vi "Update Method Accessors.vi"(8 "error in (no error)":errorcluster, 10 "RPC Method Parameters":T1, 11 "Server class in":refnum<vi>) -> (0 "error out":errorcluster, 3 "Server class out":refnum<vi>)   [LabVIEW 2019, in "gRPC Scripting Tools.lvlib"]
uses:
  gRPC Scripting Tools.lvlib
  TypeDefs/RPC Method Parameters.ctl
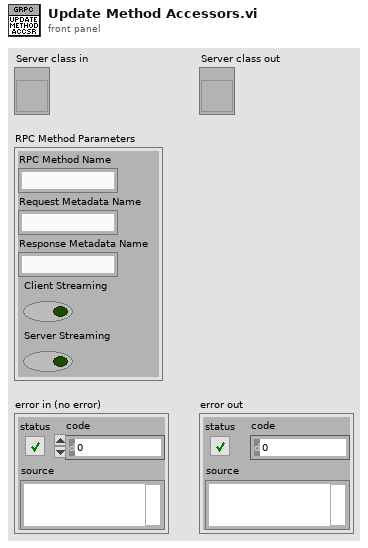
[diagram p1: front panel]
types:
  T1 = typedef "gRPC Scripting Tools.lvlib/RPC Method Parameters.ctl" = cluster{"RPC Method Name":string, "Request Metadata Name":string, "Response Metadata Name":string, "Client Streaming":bool, "Server Streaming":bool}
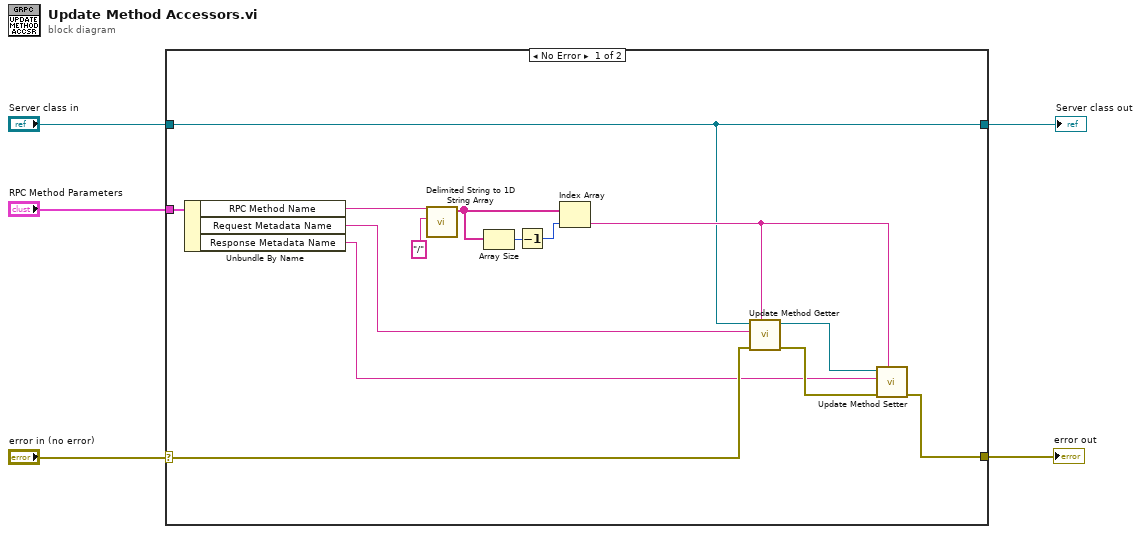
[diagram p0: block diagram]
diagram:
  n1 = case shown="No Error" "error in (no error)" {
    selector: "error in (no error)" -> [w12 w20]
    tunnel: "RPC Method Parameters" -> [w19 _]
    tunnel: "Server class in" -> [w6 w21]
    tunnel: [w6 w21] -> w2
    tunnel: [w7 w20] -> w1
    frame No Error {
      n2 = Unbundle By Name(w19) -> ("RPC Method Name"=w14:string, "Request Metadata Name"=w13:string, "Response Metadata Name"=w8:string)
      n3 = call <vilib>:"Delimited String to 1D String Array.vi"("delimiter"="/", "delimited string"=w14) -> ("string array"=w18:string[])  [unwired: 9 in]
      n4 = Array Size(array=w18) -> (size(s)=w16:i32)
      n5 = Decrement(x=w16) -> (x-1=w17:i32)
      n6 = Index Array(array=w18, index=w17) -> (element=w9:string)
      n7 = call "Update Method Getter.vi"("RPC Method Name"=w9, "error in (no error)"=w12, "Request Metadata Name"=w13, "Server class in"=w6) -> ("error out"=w11:errorcluster, "Server class out"=w10:refnum<vi>)  [unwired: 6 in]
      n8 = call "Update Method Setter.vi"("RPC Method Name"=w9, "error in (no error)"=w11, "Response Metadata Name"=w8, "Server class in"=w10) -> ("error out"=w7:errorcluster)  [unwired: 6 in, 1 out]
    }
    frame Error {
    }
  }
  "error out" <- w1
  "Server class out" <- w2
